vi "mouse_direction.vi"(0 "CtlRef":refnum<vi>, 7 "direction":enum16{"enter", "leave"}(ring), 9 "enterColors":cluster{u32, u32}[](array[cluster])=[{15830062, 15830062}, {15830062, 15830062}, {15830062, 15830062}, {14122281, 14122281}], 11 "leaveColors":cluster{u32, u32}[](array[cluster])=[{3100273, 3100273}, {15830062, 15830062}]) -> ()   [LabVIEW 2017]
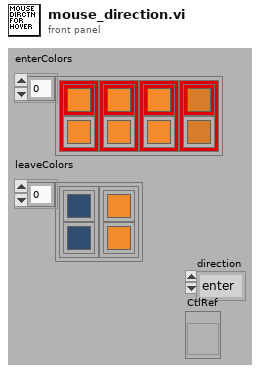
[diagram p1: front panel]
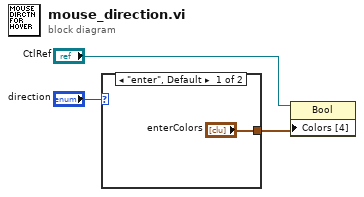
[diagram p0: block diagram]
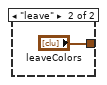
[diagram p2: hidden frame]
diagram:
  n1 = case shown="\"enter\", Default" "direction" {
    tunnel: ["enterColors" "leaveColors"] -> w1
    frame "enter", Default {
    }
    frame "leave" {
    }
  }
  n2 = property class="Bool"(reference="CtlRef", "Colors [4]"=w1) -> ()  [unwired: 1 in, 2 out]
